vi "SNMP Get Random Port Number.vi"(8 "error in (no error)":errorcluster, 9 "Maximum Port Number":u16=32767 min=1024 max=32767 step=1, 10 "Minimum Port Number":u16=1024 min=1024 max=32767 step=1) -> (0 "error out":errorcluster, 2 "UDP Port":u16, 3 "connection ID":refnum<k16>)   [LabVIEW 2017]
doc: "This VI is used to open a port for the SNMP driver. It will use a random port number and attempt to establish a port 10 times. It will return a error if it is unable to open a port after the 10 attempts."
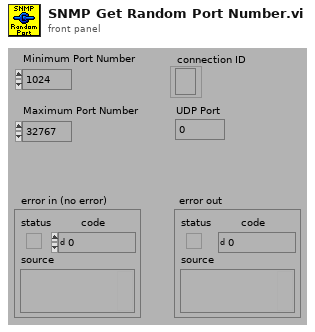
[diagram p1: front panel]
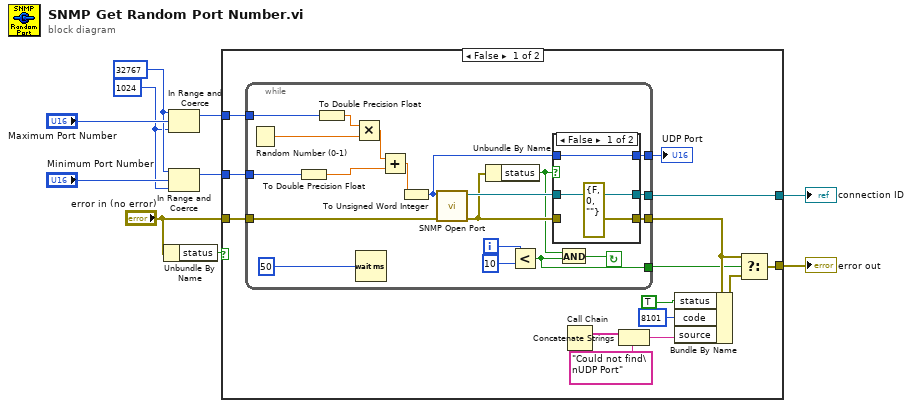
[diagram p0: block diagram]
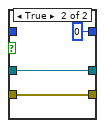
[diagram p2: hidden frame]
diagram:
  w4 = u16 32767
  w3 = u16 1024
  n1 = Unbundle By Name("error in (no error)") -> ("status"=w1:bool)
  n2 = In Range and Coerce(upper limit=w4, x="Maximum Port Number", lower limit=w3) -> (coerced(x)=w5:u16)  [unwired: 1 out]
  n3 = In Range and Coerce(upper limit=w4, x="Minimum Port Number", lower limit=w3) -> (coerced(x)=w8:u16)  [unwired: 1 out]
  n4 = case shown="False" w1 {
    tunnel: [w16 w51] -> w10
    tunnel: "error in (no error)" -> [w15 w51]
    tunnel: [w14 _] -> w9
    tunnel: w8 -> [w12 _]
    tunnel: w5 -> [w11 _]
    frame False {
      n5 = while {
        tunnel: w11 -> [w25]
        tunnel: w12 -> [w26]
        tunnel: [w27] -> w13
        tunnel: [w31] -> w17
        tunnel: [w37] -> w24
        tunnel: w15 -> [w44]
        tunnel: [w39] -> w14
        i -> [w36]
        stop <- w32 continue-if-true
        n6 = Random Number (0-1)() -> (number: 0 to 1=w43:dbl)
        n7 = To Double Precision Float(number=w26) -> (double precision float=w29:dbl)
        n8 = To Double Precision Float(number=w25) -> (double precision float=w30:dbl)
        n9 = Multiply(x=w30, y=w43) -> (x*y=w42:dbl)
        n10 = Wait (ms)(milliseconds to wait=u32 50) -> ()  [unwired: 1 out]
        n11 = Add(x=w42, y=w29) -> (x+y=w41:dbl)
        n12 = To Unsigned Word Integer(number=w41) -> (unsigned 16bit integer=w28:u16)
        n13 = call "SNMP Open Port.vi"("error in (no error)"=w44, "port"=w28) -> ("error out"=w38:errorcluster, "connection ID"=w40:refnum<k16>)  [unwired: 8 out]
        n14 = Unbundle By Name(w38) -> ("status"=w33:bool)
        n15 = Less?(x=w36, y=10) -> (x < y?=w31:bool)
        n16 = case shown="False" w33 {
          tunnel: w40 -> [w46 w50]
          tunnel: [w46 w50] -> w39
          tunnel: w38 -> [_ w49]
          tunnel: [errorcluster {"status"=FALSE, "code"=0, "source"=""} ("error out") w49] -> w37
          tunnel: w28 -> [w45 _]
          tunnel: [w45 u16 0] -> w27
          frame False {
          }
          frame True {
          }
        }
        n17 = And(x=w33, y=w31) -> (x .and. y?=w32:bool)
      }
      "UDP Port" <- w13
      n18 = Call Chain() -> (call chain=w18:string[])
      n19 = Concatenate Strings(w18, "Could not find\nUDP Port" ("Substring")) -> (w20:string)
      n20 = Bundle By Name(cluster=w24, "status"=TRUE ("Bundle Element"), "code"=8101 ("Bundle Element"), "source"=w20) -> (w23:errorcluster)
      n21 = Select(t=w24, s=w17, f=w23) -> (s? t:f=w16:errorcluster)
    }
    frame True {
    }
  }
  "error out" <- w10
  "connection ID" <- w9
